vi "simx Get Vision Sensor Image.vi"(0 "clientID":i32, 1 "options":u8, 5 "sensorHandle":i32, 7 "resolution":i32, 9 "image":string, 11 "error in (no error)":errorcluster, 12 "operationMode":i32) -> (4 "function return":i32, 8 "resolution out":i32, 10 "image out":string, 15 "error out":errorcluster)   [LabVIEW 2019, in "PXL_V-REP.lvlib"]
doc: "EXTAPI_DLLEXPORT simxInt simxGetVisionSensorImage(simxInt clientID,simxInt sensorHandle,simxInt* resolution,simxUChar** image,simxUChar options,simxInt operationMode);"
uses:
  PXL_V-REP.lvlib
  <userlib>/V-REP/remoteApi.dll
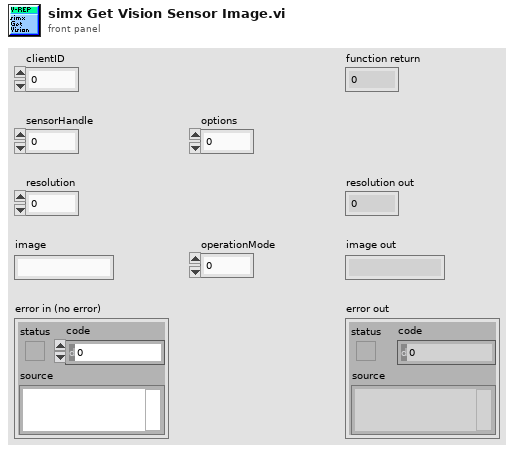
[diagram p1: front panel]
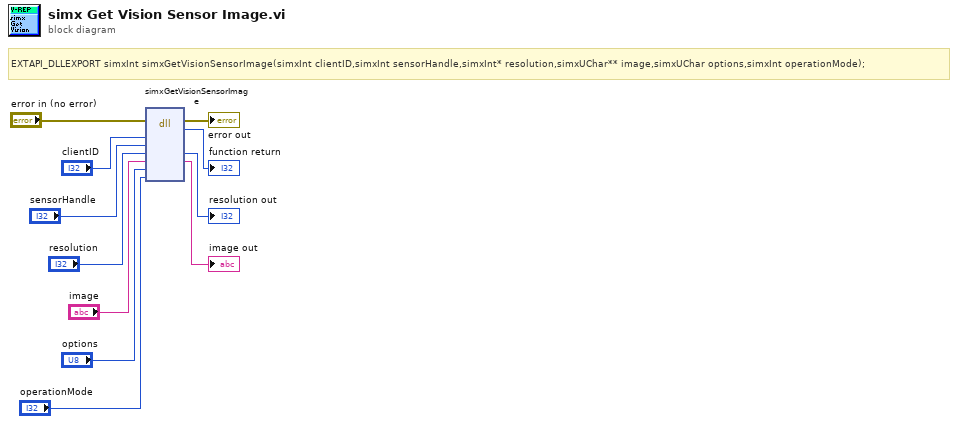
[diagram p0: block diagram]
diagram:
  # "EXTAPI_DLLEXPORT simxInt simxGetVisionSensorImage(simxInt clientID,simxInt sensorHandle,simxInt* resolution,simxUChar** image,simxUChar options,simxInt operationMode);"
  n1 = dll-call lib="C:/Program Files (x86)/National Instruments/LabVIEW 2019/user.lib/V-REP/remoteApi.*" fn="simxGetVisionSensorImage"(error in="error in (no error)", "clientID"="clientID", "sensorHandle"="sensorHandle", "resolution"="resolution", "image"="image", "options"="options", "operationMode"="operationMode") -> (error out=→"error out":errorcluster, →"function return":i32, "resolution"=→"resolution out":i32, "image"=→"image out":string)  [unwired: 6 in, 1 out]
